vi "Current - Continuous Input - LazyWave.vi"(8 "Tempo Aquisicao":dbl=120.0, 9 "TDMS File Path":path=path "C:/Users/Adquiri/Downloads/Adquiri_LazyWave/Aquisicao/Dados/Novo Documento de Texto.tdms", 10 "Sample Rate":dbl=3000.0, 11 "task/channels in":refnum<k21>="ADQUIRE") -> ()   [LabVIEW 2019]
doc: "This example demonstrates how to continuously acquire buffered current measurements using a DAQmx device.\n\nFor instructions on how to connect your signals to the DAQ device, refer to your device documentation."
uses:
  <vilib>/Utility/error.llb/DialogType.ctl
  <vilib>/DAQmx/read.llb/DAQmx Read (Analog 2D DBL NChan NSamp).vi
  <vilib>/DAQmx/configure/timing.llb/DAQmx Timing (Sample Clock).vi
  <vilib>/DAQmx/configure/task.llb/DAQmx Configure Logging (TDMS).vi
  <vilib>/DAQmx/miscellaneous.llb/DAQmx Fill In Error Info.vi
  <resource>/objmgr/daqmx.rc
panel:
  out "Time":i32
  in  "Stop":bool
  out "Waveform Graph":dbl[][](graph)
  out "Actual Sample Rate":dbl=1000.0 format="%0.2f"
  # "Channel Settings"
  # "Acquired Data"
  # "Timing Settings"
  # "[s]"
  # "Aquisition Settings"
  # "Logging Settings"
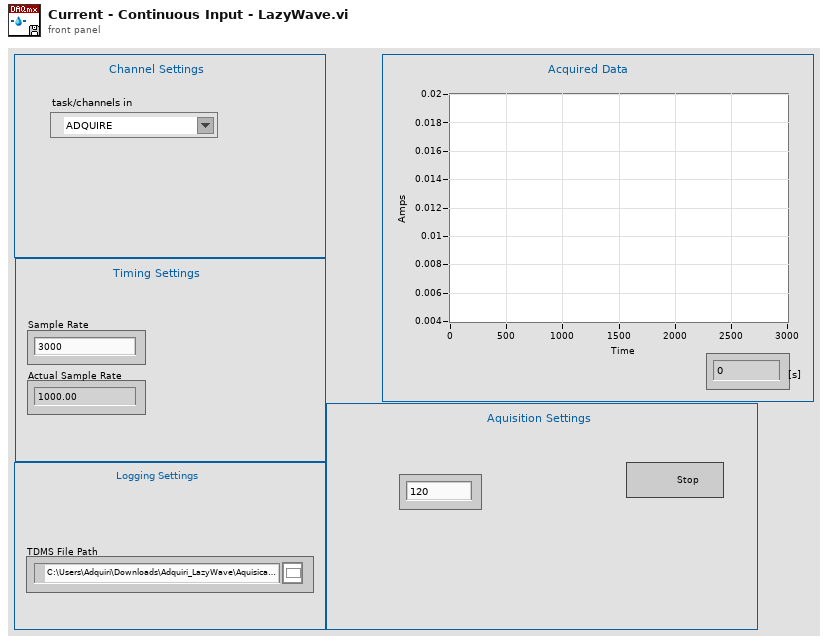
[diagram p1: front panel]
types:
  T1 = typedef "DialogType.ctl" = u16
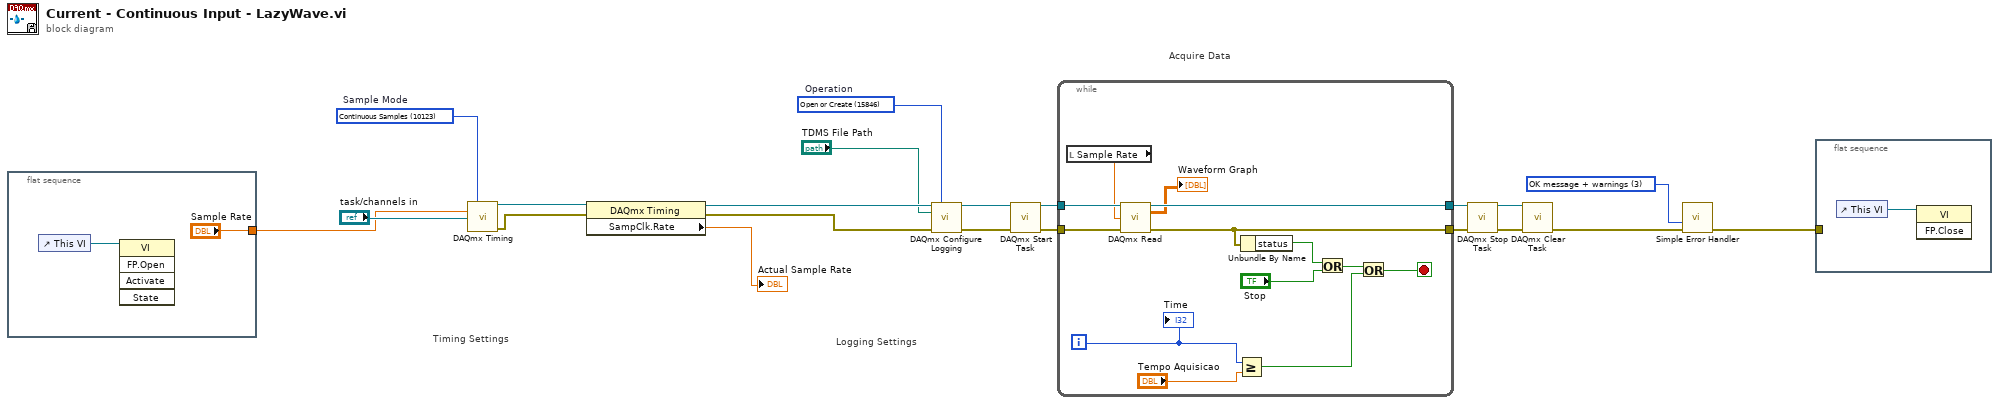
[diagram p0: block diagram]
diagram:
  w6 = T1 3 items=["no dialog", "OK message", "continue or stop message", "OK message + warnings", "continue/stop + warnings"] ("type of dialog (OK msg:1)")
  w16 = 15846 items=["Open"=10437, "Open or Create"=15846, "Create or Replace"=15847, "Create"=15848]  # Operation
  w19 = 10123 items=["Finite Samples"=10178, "Continuous Samples"=10123, "Hardware Timed Single Point"=12522]  # Sample Mode
  # "Acquire Data"
  # "Timing Settings"
  # "Logging Settings"
  n1 = flat-sequence {
    tunnel: ["Sample Rate"] -> w1
    frame #0 {
      n2 = control-ref of="This VI"() -> (w23:refnum<vi>)
      n3 = invoke class="VI" method="FP.Open"(reference=w23) -> ()  [unwired: 4 in, 5 out]
    }
  }
  n4 = call-poly <vilib>:"DAQmx Timing.vi"("task/channels in"="task/channels in", "sample mode"=w19, "rate"=w1) -> ("task out"=w21:refnum<k21>, "error out"=w20:errorcluster)  [unwired: 11 in]
  n5 = property class="DAQmx Timing"(reference=w21, error in=w20) -> (reference out=w18:refnum<k21>, error out=w17:errorcluster, "SampClk.Rate"=→"Actual Sample Rate":dbl)
  n6 = call-poly <vilib>:"DAQmx Configure Logging.vi"("task/channels in"=w18, "operation"=w16, "file path"="TDMS File Path", "error in"=w17) -> ("task out"=w4:refnum<k21>, "error out"=w3:errorcluster)  [unwired: 10 in]
  n7 = call <vilib>:"DAQmx Start Task.vi"("task/channels in"=w4, "error in"=w3) -> ("task out"=w15:refnum<k21>, "error out"=w14:errorcluster)  [unwired: 12 in]
  n8 = while {
    tunnel: w15 -> [w36]
    tunnel: w14 -> [w35]
    tunnel: [w33] -> w9
    tunnel: [w34] -> w10
    i -> [w29]
    stop <- w25 stop-if-true
    n9 = local read "Sample Rate"() -> (w24:dbl)
    n10 = call-poly <vilib>:"DAQmx Read.vi"("task/channels in"=w36, "number of samples per channel"=w24, "error in"=w35) -> ("task out"=w34:refnum<k21>, "data"=→"Waveform Graph":dbl[][], "error out"=w33:errorcluster)  [unwired: 10 in]
    n11 = Greater Or Equal?(x=w29, y="Tempo Aquisicao") -> (x >= y?=w27:bool)
    n12 = Unbundle By Name(w33) -> ("status"=w32:bool)
    n13 = Or(x=w32, y="Stop") -> (x .or. y?=w26:bool)
    n14 = Or(x=w26, y=w27) -> (x .or. y?=w25:bool)
    "Time" <- w29
  }
  n15 = call <vilib>:"DAQmx Stop Task.vi"("task/channels in"=w10, "error in"=w9) -> ("task out"=w8:refnum<k21>, "error out"=w7:errorcluster)  [unwired: 12 in]
  n16 = call <vilib>:"DAQmx Clear Task.vi"("task in"=w8, "error in"=w7) -> ("error out"=w13:errorcluster)  [unwired: 13 in]
  n17 = call <vilib>:"Simple Error Handler.vi"("type of dialog (OK msg:1)"=w6, "error in (no error)"=w13) -> ("error out"=w2:errorcluster)  [unwired: 3 in, 4 out]
  n18 = flat-sequence {
    tunnel: w2 -> [_]
    frame #0 {
      n19 = control-ref of="This VI"() -> (w37:refnum<vi>)
      n20 = invoke class="VI" method="FP.Close"(reference=w37) -> ()  [unwired: 2 in, 3 out]
    }
  }
